vi "Day-02 pt 1 Submarine Navigation.vi"() -> ()   [LabVIEW 2020, in "Advent of Code.lvlib"]
uses:
  Advent of Code.lvlib
panel:
  in  "Input":string="forward 5\nforward 1\nforward 3\ndown 8\nup 6\ndown 5\nforward 6\ndown 9\ndown 7\nup 9\ndown 9\nforward 5\nforward 3\ndown 3\nforward 1\nforward 8\ndown 8\nforward 6\nforward 9\nforward 5\ndown 8\nup 1\nforward 4\nforward 8\ndown 4\nforward 2\ndown 1\nup 8\nup 9\ndown 4\nforward 5\nup 9\nforward 1\ndown 9\ndown 7\ndown 4\ndown 6\ndown 3\nforward 5\nup 4\nup 7\nforward 1\ndown 1\nup 3\nforward 8\ndown 8\nup 2\nforward 2\ndown 7\ndown 7\ndown 4\nforward 3\ndown 5\nup 8\ndown 6\nup 2\ndown 7\nforward 8\ndown 7\ndown 7\nup 6\nforward 8\nup 1\ndown 4\nforward 1\ndown 1\ndown 9\ndown 1\ndown 7\nforward 2\nforward 3\nup 8\nup 1\nforward 4\nforward 7\nforward 9\nup 8\ndown 9\ndown 3\ndown 5\ndown 5\nforward 7\nforward 3\nup 7\nforward 6\nup 6\nforward 3\ndown 2\ndown 5\ndown 2\nup 6\ndown 5\ndown 5\nforward 7\nforward 2\nforward 7\ndown 6\nforward 1\nforward 8\nup 6\nforward 2\ndown 5\nforward 3\nup 2\nforward 3\ndown 2\nforward 4\nforward 6\ndown 8\nforward 7\nforward 6\ndown 1\ndown 8\nforward 7\nup 2\nforward 2\ndown 7\nup 6\nforward 7\ndown 9\ndown 7\nforward 4\ndown 9\ndown 4\nforward 6\nup 6\nup 5\ndown 5\nup 7\nforward 6\ndown 1\ndown 5\nforward 1\nup 6\nforward 1\ndown 7\nforward 7\nforward 4\nup 5\ndown 3\nforward 7\nforward 6\nup 9\nforward 8\nforward 1\nup 2\nup 8\nforward 7\nup 7\ndown 1\nforward 9\ndown 5\nforward 5\nforward 2\nforward 2\nforward 6\nup 5\nup 1\nforward 6\nup 3\ndown 7\ndown 6\ndown 1\nforward 1\nforward 8\nforward 8\ndown 8\nup 3\ndown 7\ndown 2\ndown 9\nforward 9\ndown 7\nforward 4\ndown 9\nforward 8\ndown 1\ndown 5\ndown 9\ndown 8\nforward 8\ndown 3\nforward 4\nforward 6\nup 3\nforward 4\ndown 9\ndown 6\nup 6\nup 3\ndown 2\nup 1\nforward 5\ndown 7\ndown 3\nforward 5\nup 1\nforward 2\ndown 3\ndown 3\nforward 6\ndown 5\ndown 7\ndown 1\ndown 2\ndown 7\nforward 4\nforward 7\ndown 7\nforward 6\nforward 2\ndown 1\ndown 8\nforward 5\nforward 5\ndown 7\nforward 6\nforward 7\nup 2\nforward 5\ndown 8\nforward 7\ndown 7\nup 6\nforward 6\ndown 2\ndown 7\nforward 6\nforward 4\ndown 5\ndown 7\nforward 2\nforward 6\nforward 6\ndown 7\ndown 9\nforward 9\nforward 4\nup 9\nup 2\nup 2\nforward 4\ndown 6\nforward 7\nup 5\nforward 1\nforward 6\ndown 8\nforward 2\ndown 8\nforward 9\nforward 5\nforward 1\nup 8\ndown 4\ndown 2\ndown 9\nup 6\nforward 8\ndown 9\nforward 3\ndown 3\ndown 9\ndown 9\ndown 6\nforward 7\ndown 4\nforward 8\ndown 7\ndown 8\nup 4\nup 3\nforward 1\nup 9\nup 1\nup 9\nup 7\ndown 1\nforward 5\nforward 7\nforward 3\nforward 8\nup 4\nforward 7\ndown 5\nforward 9\nup 3\nup 3\ndown 2\nforward 3\nup 3\ndown 3\ndown 4\nup 6\ndown 7\ndown 1\ndown 7\nforward 1\ndown 4\nforward 9\ndown 9\nup 8\nup 5\ndown 7\nup 1\nforward 6\ndown 1\ndown 4\ndown 3\nforward 7\nforward 4\nup 6\ndown 2\ndown 1\nforward 1\nup 5\ndown 2\ndown 9\nup 2\nup 3\nforward 5\nforward 5\ndown 8\ndown 4\nup 4\ndown 1\nforward 8\nup 7\ndown 1\ndown 4\nforward 3\nup 4\ndown 4\ndown 5\ndown 9\ndown 1\ndown 7\nup 2\ndown 6\nup 9\ndown 3\ndown 1\ndown 8\ndown 4\nup 2\nforward 6\nforward 9\ndown 6\nforward 6\nforward 4\nforward 8\nforward 5\nforward 6\nforward 9\ndown 3\nforward 8\nforward 6\nforward 7\nup 9\nforward 3\nup 3\nforward 5\ndown 5\nup 9\nforward 1\nforward 9\ndown 7\nforward 5\nforward 5\nforward 6\nforward 5\nforward 9\nforward 8\nforward 3\ndown 2\nforward 6\nforward 8\ndown 4\nforward 4\nforward 1\nforward 1\ndown 2\nforward 2\nforward 5\nup 4\nforward 3\ndown 3\ndown 5\ndown 6\nforward 4\ndown 8\ndown 4\nforward 5\ndown 7\nup 3\nup 6\nforward 3\nforward 2\nforward 5\ndown 9\ndown 4\ndown 8\ndown 2\nforward 4\nforward 7\ndown 4\nup 5\nforward 8\ndown 8\ndown 1\nforward 5\ndown 6\ndown 9\nup 6\nforward 9\ndown 3\nforward 6\nforward 2\ndown 5\nforward 1\ndown 1\ndown 1\nforward 2\nup 9\ndown 1\nup 8\nforward 9\nup 8\nforward 2\nforward 8\nup 2\nforward 4\ndown 5\nforward 8\nup 2\nup 1\nforward 4\nup 4\nup 3\nup 5\ndown 1\nforward 3\nforward 6\nforward 9\nforward 6\nup 8\nforward 2\nforward 1\ndown 2\ndown 3\ndown 2\nup 4\nforward 5\nup 2\nforward 3\nforward 9\nup 5\nforward 1\ndown 7\nforward 9\ndown 5\nup 7\ndown 6\nforward 7\nforward 9\nup 6\nforward 3\ndown 1\nforward 1\ndown 8\ndown 2\nup 9\ndown 4\ndown 4\ndown 7\nforward 4\nforward 1\nforward 6\ndown 9\ndown 9\ndown 9\nforward 1\nforward 6\nforward 3\nforward 7\nforward 3\nforward 9\nup 8\nforward 5\ndown 1\ndown 6\nup 8\nforward 3\nup 8\ndown 6\nforward 6\nup 2\nup 8\nup 5\nforward 9\ndown 4\nup 1\nup 3\nup 2\ndown 9\ndown 1\nforward 7\ndown 2\nforward 6\nup 4\ndown 7\nforward 1\ndown 3\ndown 5\nforward 1\ndown 3\ndown 1\nforward 8\nup 5\nforward 5\nforward 8\nforward 8\nforward 8\nforward 2\ndown 3\ndown 6\nup 2\nup 2\ndown 1\nup 7\ndown 9\nup 1\nup 4\nforward 1\nforward 4\nup 4\nup 6\nforward 5\nforward 2\nforward 7\nup 8\nup 3\ndown 5\ndown 9\nforward 4\nforward 5\nforward 5\ndown 1\nup 8\nup 2\nforward 3\nup 2\nforward 8\nup 2\ndown 6\nup 7\nforward 6\ndown 3\nforward 3\ndown 6\nforward 6\nforward 4\nforward 8\ndown 8\nup 7\ndown 7\ndown 2\nup 5\nup 2\ndown 4\nforward 5\ndown 3\nup 4\ndown 2\nup 2\ndown 7\nforward 4\nforward 3\nforward 6\ndown 2\ndown 8\nforward 3\nforward 4\nforward 4\ndown 4\ndown 3\nup 6\ndown 2\nforward 7\nforward 4\ndown 7\nforward 1\nup 6\nforward 3\nup 3\nup 7\nforward 6\ndown 9\ndown 8\ndown 3\nforward 8\nforward 1\nup 3\ndown 5\ndown 3\nforward 1\nup 9\ndown 6\nforward 3\ndown 9\nup 7\nforward 5\nforward 4\nforward 7\nup 3\nforward 3\ndown 5\nforward 7\nforward 9\ndown 6\nforward 7\nforward 5\nup 6\nforward 3\nforward 3\ndown 7\nforward 4\nup 2\nforward 8\ndown 7\nup 7\ndown 7\nforward 6\nup 3\nforward 2\nup 7\ndown 3\ndown 4\ndown 1\nforward 3\nforward 5\nup 7\nforward 3\ndown 1\ndown 2\nup 4\nforward 2\nup 5\ndown 4\nforward 1\ndown 6\nup 1\nforward 5\nforward 1\ndown 8\nforward 7\ndown 7\nforward 4\nforward 7\nforward 3\nforward 2\nforward 1\nforward 7\ndown 1\nforward 9\nforward 9\nforward 8\nforward 9\nforward 8\nforward 5\nforward 1\nup 5\nforward 3\nforward 6\nforward 1\nup 4\ndown 1\ndown 9\ndown 6\nforward 4\nup 9\ndown 3\nforward 2\ndown 3\nup 2\nforward 4\nforward 4\ndown 7\nforward 9\nforward 3\ndown 4\nup 4\ndown 4\nforward 7\nforward 3\nforward 6\nforward 9\ndown 4\ndown 5\ndown 2\nforward 4\nup 6\nforward 8\nforward 3\ndown 2\ndown 5\nforward 4\ndown 8\nup 5\ndown 3\nforward 6\ndown 8\nup 9\nforward 3\nforward 8\nforward 6\nforward 7\ndown 3\nup 6\ndown 7\ndown 4\nforward 2\nforward 5\ndown 1\ndown 5\ndown 5\nforward 6\nforward 6\ndown 1\nforward 2\nup 1\ndown 2\ndown 3\nforward 3\nforward 9\ndown 9\ndown 1\nup 8\ndown 5\ndown 2\nup 7\nforward 8\nup 7\nforward 3\nforward 6\ndown 2\ndown 3\nforward 1\ndown 6\ndown 1\nforward 4\nup 2\ndown 3\nup 7\ndown 3\ndown 2\nup 8\nup 7\ndown 3\nforward 4\ndown 8\nup 2\ndown 6\nforward 9\ndown 1\nup 3\nup 1\ndown 4\nup 6\ndown 2\nforward 1\ndown 6\nforward 4\nforward 3\ndown 7\ndown 2\ndown 6\ndown 2\ndown 7\nforward 2\ndown 1\nup 8\nup 6\nup 1\nforward 5\ndown 9\ndown 5\nup 7\ndown 4\nforward 4\nforward 5\nup 5\nforward 6\nforward 1\nforward 5\nforward 1\nforward 6\ndown 6\nforward 3\nup 4\nforward 6\ndown 6\nforward 1\nforward 5\nforward 8\ndown 3\nforward 6\nforward 1\nup 1\nup 7\nforward 7\nforward 8\nup 6\nforward 9\nup 5\nforward 1\nforward 5\ndown 3\nup 3\nup 9\nforward 9\nforward 5\nforward 3\nforward 2\nforward 4\ndown 6\nup 5\ndown 2\nforward 5\ndown 2\ndown 5\ndown 6\nforward 7\ndown 2\nforward 7\nforward 2\nforward 8\nup 1\nforward 9\ndown 2\nup 1\ndown 9\nforward 8\nforward 3\nup 9\ndown 1\ndown 1\ndown 8\nup 4\nup 9\nforward 9\nforward 3\ndown 9\nforward 3\nforward 4\ndown 8\nforward 8\nforward 7\ndown 9\nup 2\ndown 9\ndown 8\ndown 9\nforward 4\nup 6\ndown 4\nforward 8\nforward 5\nup 2\nforward 5\ndown 3\nforward 6\ndown 5\nforward 8\nup 3\ndown 5\ndown 4\nforward 5\nup 3\nup 8\nforward 1\nup 8\nforward 4\ndown 4\nforward 7\nforward 5\nforward 7\nforward 9\nup 1\ndown 6\nforward 8\nup 1\ndown 5\nup 6\ndown 9\ndown 5\nforward 3\nup 1\nforward 4\nup 4\ndown 4\nforward 5\nforward 8\ndown 2\nup 7\ndown 6\nforward 7\nup 7\nforward 5\ndown 2\nforward 9\nforward 1\ndown 9\ndown 8\nforward 7\nforward 7\nforward 1\nup 3\nup 1\nforward 2\ndown 2\nup 9\ndown 2\nforward 7\ndown 1\ndown 5\ndown 4\nup 7\nforward 1\ndown 3\nforward 9\ndown 6\nforward 4\ndown 4\ndown 9\ndown 3\nup 3\ndown 3\nup 8\ndown 2\nforward 1\nforward 5\nforward 5\ndown 2\nforward 7\ndown 7\ndown 6\nforward 6\nup 5\ndown 4\ndown 8\ndown 7\nforward 7\nup 3\ndown 3\ndown 3\nforward 8\nforward 5\ndown 1\nup 6\ndown 3\nup 2\ndown 6\nup 7\ndown 4\nup 2\nforward 4\nforward 9\nforward 9\nup 1\nforward 7\nup 7\nforward 7\nforward 6\nforward 3\nforward 1\ndown 5\ndown 3\nforward 4\nup 9\ndown 5\nup 2\ndown 6\ndown 5\nforward 6\nforward 4\nup 7\nup 6\ndown 9\nforward 4\nup 1\nup 6\nup 3\nforward 9\nforward 3\nforward 9\ndown 7\nforward 6\ndown 6\nforward 8"
  out "Displacement Product":i32
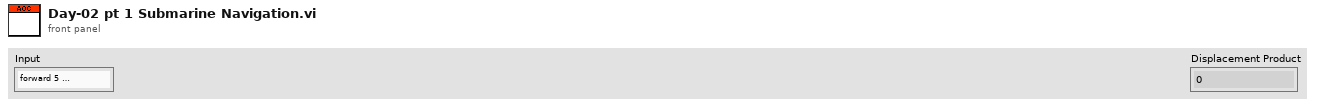
[diagram p1: front panel]
types:
  T1 = typedef "Advent of Code.lvlib/Navigation Command.ctl" = cluster{"Direction":T2, "Value":i32}
  T2 = typedef "Advent of Code.lvlib/Navigation Directions.ctl" = enum16{"forward", "down", "up"}
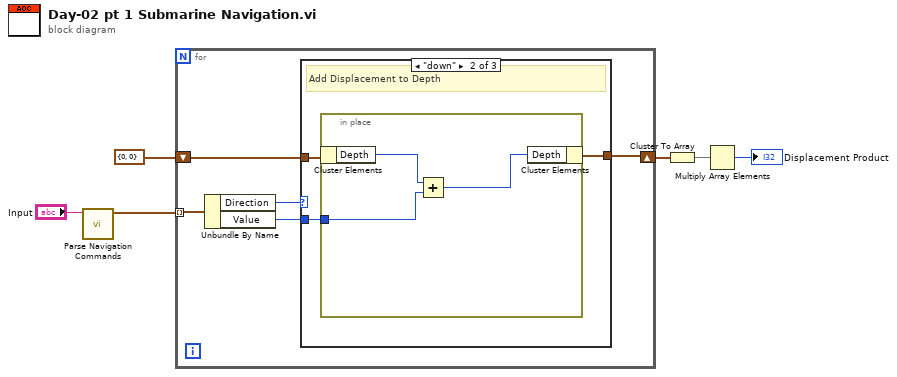
[diagram p0: block diagram]
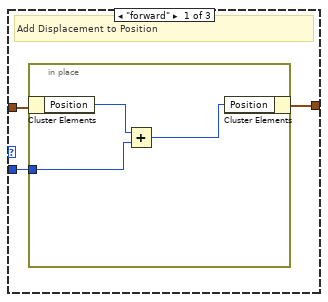
[diagram p2: hidden frame]
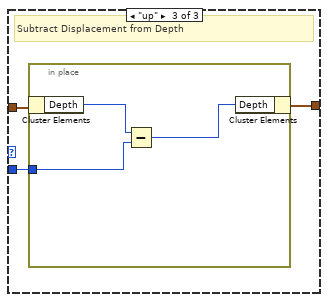
[diagram p3: hidden frame]
diagram:
  n1 = call "Parse Navigation Commands.vi"("Input"="Input") -> ("Commands"=w5:T1[])  [unwired: 9 in, 1 out]
  n2 = for {
    tunnel: w5 -> [w11] mode=indexing
    shift-right: [w7] -> w3
    shift-left: cluster{"Depth":i32, "Position":i32} {"Depth"=0, "Position"=0} -> [w8]
    n3 = Unbundle By Name(w11) -> ("Direction"=w10:T2, "Value"=w9:i32)
    n4 = case shown="\"down\"" w10 {
      tunnel: w9 -> [w13 w19 w25]
      tunnel: w8 -> [w14 w20 w26]
      tunnel: [w12 w18 w24] -> w7
      frame "forward" {
        # "Add Displacement to Position"
        n5 = in-place {
          in-place-border: w13 -> [w17]
          n6 = in-place-cluster #1(w14) -> ("Position"=w16:i32)
          n7 = Add(x=w16, y=w17) -> (x+y=w15:i32)
          n8 = in-place-cluster #1("Position"=w15) -> (w12:cluster{"Depth":i32, "Position":i32})
        }
      }
      frame "down" {
        # "Add Displacement to Depth"
        n9 = in-place {
          in-place-border: w19 -> [w23]
          n10 = in-place-cluster #2(w20) -> ("Depth"=w22:i32)
          n11 = Add(x=w22, y=w23) -> (x+y=w21:i32)
          n12 = in-place-cluster #2("Depth"=w21) -> (w18:cluster{"Depth":i32, "Position":i32})
        }
      }
      frame "up" {
        # "Subtract Displacement from Depth"
        n13 = in-place {
          in-place-border: w25 -> [w29]
          n14 = in-place-cluster #3(w26) -> ("Depth"=w28:i32)
          n15 = Subtract(x=w28, y=w29) -> (x-y=w27:i32)
          n16 = in-place-cluster #3("Depth"=w27) -> (w24:cluster{"Depth":i32, "Position":i32})
        }
      }
    }
  }
  n17 = Cluster To Array(cluster=w3) -> (array=w2:i32[])
  n18 = Multiply Array Elements(1:w2) -> (0:→"Displacement Product":i32)
